vi "lab_3_4.vi"() -> ()   [LabVIEW 2014]
uses:
  <vilib>/addons/Multicore Analysis and Sparse Matrix/Statistics/_statistics/Mean (DBL).vi
  <vilib>/measure/NI_MABase.lvlib
  <vilib>/addons/Multicore Analysis and Sparse Matrix/Statistics/NI_MASM_Statistics.lvlib
panel:
  in  "sampling info":cluster{"Fs":dbl, "#s":dbl}={"Fs"=1000.0, "#s"=1000.0} {"Fs" format="%.2p"}
  in  "tempo tot acquisiz":dbl
  in  "durata ciclo\n acquisizione dt":dbl
  in  "freq acquiisizione":dbl
  out "XY Graph":cluster{dbl[], dbl[]}(graph)
  in  "freq quadra":dbl=10.0 format="%0.2p"
  in  "amp quadra":dbl=1.0 format="%0.2p"
  out "Waveform Graph 2":waveform(dbl)(graph)
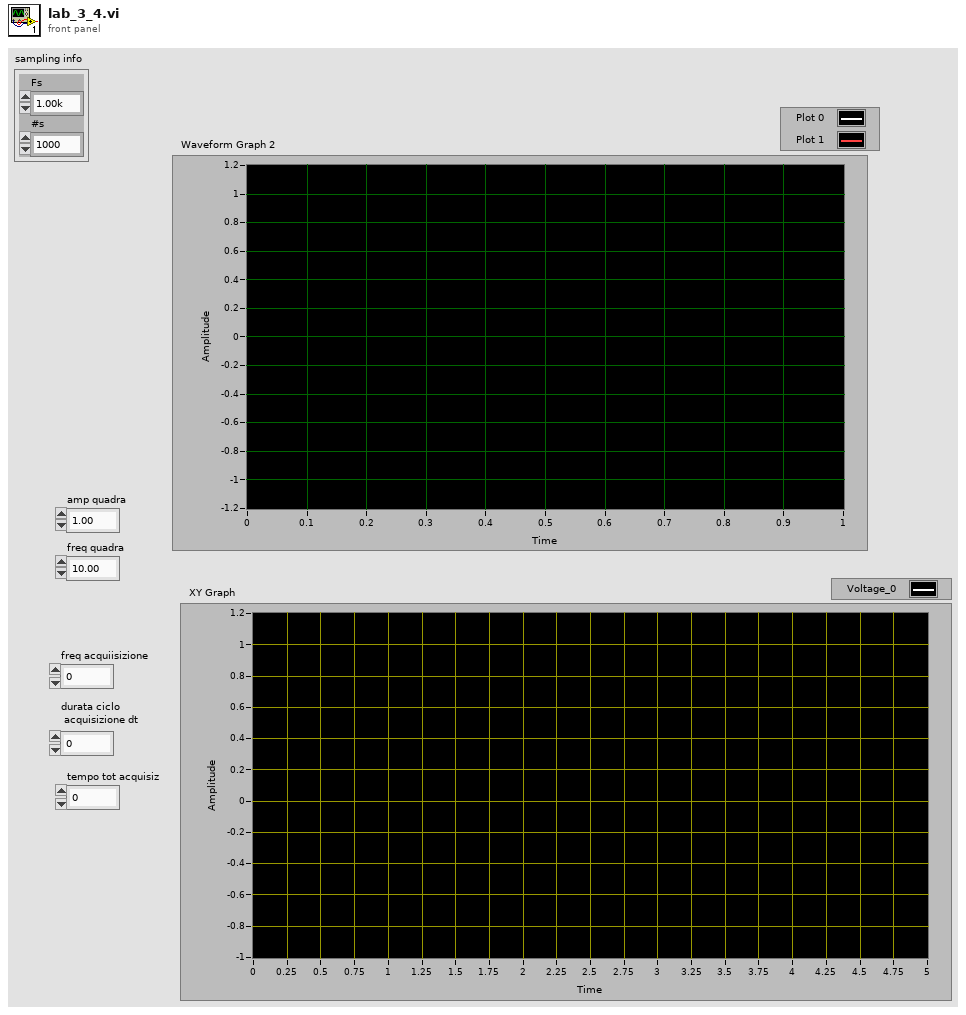
[diagram p1: front panel]
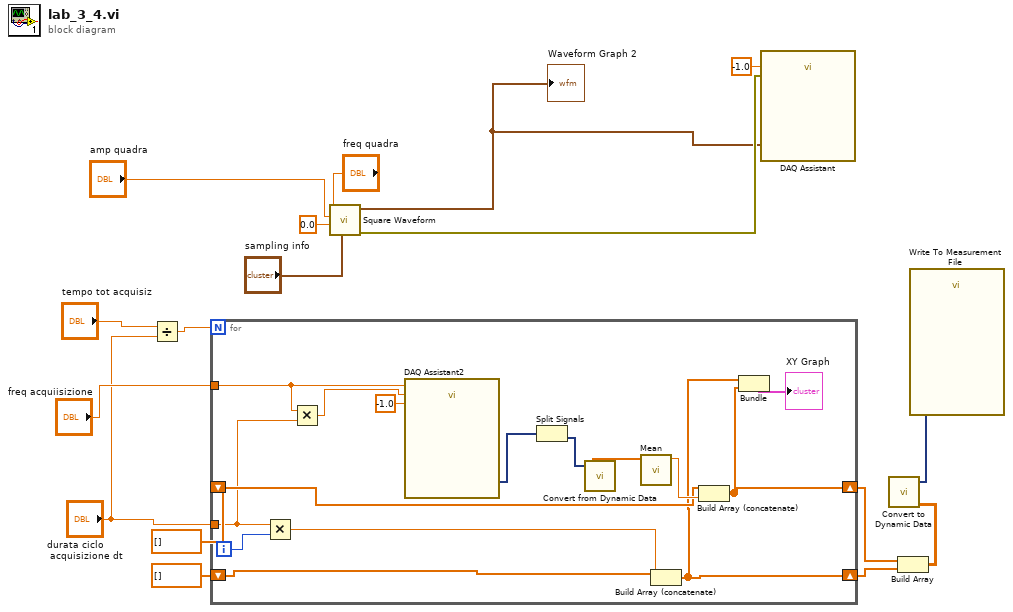
[diagram p0: block diagram]
diagram:
  n1 = Divide(x="tempo tot acquisiz", y="durata ciclo\n acquisizione dt") -> (x/y=w13:dbl)
  n2 = for {
    N: w13 -> [_]
    shift-right: [w21] -> w10
    shift-left: dbl[] [] -> [w29]
    tunnel: "durata ciclo\n acquisizione dt" -> [w23]
    shift-right: [w20] -> w9
    shift-left: dbl[] [] -> [w26]
    tunnel: "freq acquiisizione" -> [w24]
    i -> [w28]
    n3 = Multiply(x=w23, y=w28) -> (x*y=w27:dbl)
    n4 = Multiply(x=w24, y=w23) -> (x*y=w22:dbl)
    n5 = call "DAQ Assistant2"("rate"=w24, "number of samples"=w22, "timeout (s)"=-1.0) -> ("data"=w19:dynamicdata)  [unwired: 14 in, 2 out]
    n6 = Split Signals(w19) -> (w18:dynamicdata)  [unwired: 2 in, 1 out]
    n7 = call "Convert from Dynamic Data"("Dynamic Data Type"=w18) -> ("Array"=w31:dbl[])  [unwired: 3 in]
    n8 = call-poly <vilib>:"Mean.vi"("X"=w31) -> ("mean"=w30:dbl)  [unwired: 9 in, 1 out]
    n9 = Build Array (concatenate)(w26, w27) -> (w20:dbl[])
    n10 = Build Array (concatenate)(w29, w30) -> (w21:dbl[])
    n11 = Bundle(w20, w21) -> (→"XY Graph":cluster{dbl[], dbl[]})  [unwired: 1 in]
  }
  n12 = call <vilib>:"Square Waveform.vi"("sampling info"="sampling info", "phase"=0.0, "amplitude"="amp quadra", "frequency"="freq quadra") -> ("error out"=w6:errorcluster, "signal out"=w3:waveform(dbl))  [unwired: 6 in]
  "Waveform Graph 2" <- w3
  n13 = call "DAQ Assistant"("data"=w3, "timeout (s)"=-1.0, "error in"=w6) -> ()  [unwired: 15 in, 2 out]
  n14 = Build Array(w10, w9) -> (w8:dbl[][])
  n15 = call "Convert to Dynamic Data"("2D Array"=w8) -> ("Dynamic Data Type"=w7:dynamicdata)  [unwired: 3 in]
  n16 = call "Write To Measurement File"("Signals"=w7) -> ()  [unwired: 16 in, 3 out]
